vi "Write Activate or Blackstart Msg.vi"(10 "Activate or Blackstart Msg":refnum<class "Activate or Blackstart Msg.lvclass">, 11 "Commissioning in":refnum<class "Commissioning.lvclass">) -> (3 "Commissioning out":refnum<class "Commissioning.lvclass">)   [LabVIEW 2018, in "Commissioning Actor.lvlib" / "Commissioning.lvclass"]
uses:
  Commissioning.lvclass
  Commissioning Messages/Activate or Blackstart Msg/Activate or Blackstart Msg.lvclass
  Commissioning.lvclass/Commissioning.ctl
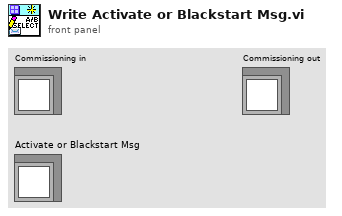
[diagram p1: front panel]
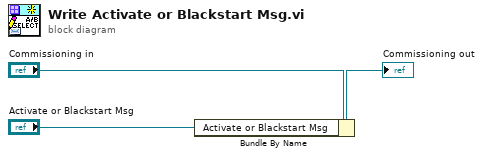
[diagram p0: block diagram]
diagram:
  n1 = Bundle By Name(cluster="Commissioning in", "Activate or Blackstart Msg"="Activate or Blackstart Msg") -> (→"Commissioning out":refnum<class "Commissioning.lvclass">)
